vi "PS-RA01B FPGA.vi"() -> ()   [LabVIEW 2011]
uses:
  <vilib>/rvi/eio/common/nirviEmuTemplateMethod_errors.vi
  <vilib>/rvi/Memory/Memory_Emulation/niFpgaMemoryEmulationValidateCache.vi
  <vilib>/rvi/DataTransferAndStorage/Container/Common/niFpgaContainerGetUniqueNameForEmu.vi
  <vilib>/rvi/Memory/Memory_Emulation/nirvimemoryEmulationManagerCache_InsertValue.vi
  <vilib>/Utility/error.llb/Clear Errors.vi
  <vilib>/rvi/Memory/Memory_Emulation/nirvimemoryEmulationManagerCache_GetValue.vi
  <vilib>/rvi/Memory/Memory_Emulation/nirvimemoryEmulationManagerCache_SetValue.vi
  <vilib>/eio/EIONode/EIONode.xnode
  <vilib>/eio/EIOMethodNode/EIOMethodNode.xnode
  <vilib>/rvi/DataTransferAndStorage/Container/XNode/niFpgaContainer.xnode
  <vilib>/rvi/Memory/Memory_Emulation/nirvimemoryEmulation.vi
panel:
  out "ADDR":u8
  out "Mod6/AO1":fxp<+/-,20,5> format="%.17g"
  out "Mod2/AO3":fxp<+/-,20,5> format="%.17g"
  out "Mod2/AO2":fxp<+/-,20,5> format="%.17g"
  out "Mod2/AO1":fxp<+/-,20,5> format="%.17g"
  out "Mod2/AO0":fxp<+/-,20,5> format="%.17g"
  out "Mod6/AO3":fxp<+/-,20,5> format="%.17g"
  out "Mod6/AO2":fxp<+/-,20,5> format="%.17g"
  out "Mod6/AO0":fxp<+/-,20,5> format="%.17g"
  out "Timestamp":u32 caption="Tick Count(Ticks)"
  out "Mod5/AI0":fxp<+/-,20,5> format="%.17g"
  out "Mod5/AI2":fxp<+/-,20,5> format="%.17g"
  out "Mod5/AI3":fxp<+/-,20,5> format="%.17g"
  out "Mod1/AI0":fxp<+/-,20,5> format="%.17g"
  out "Mod1/AI1":fxp<+/-,20,5> format="%.17g"
  out "Mod1/AI2":fxp<+/-,20,5> format="%.17g"
  out "Mod1/AI3":fxp<+/-,20,5> format="%.17g"
  out "Mod5/AI1":fxp<+/-,20,5> format="%.17g"
  out "period":u32
  out "delay":u32
  out "dperiod":u32
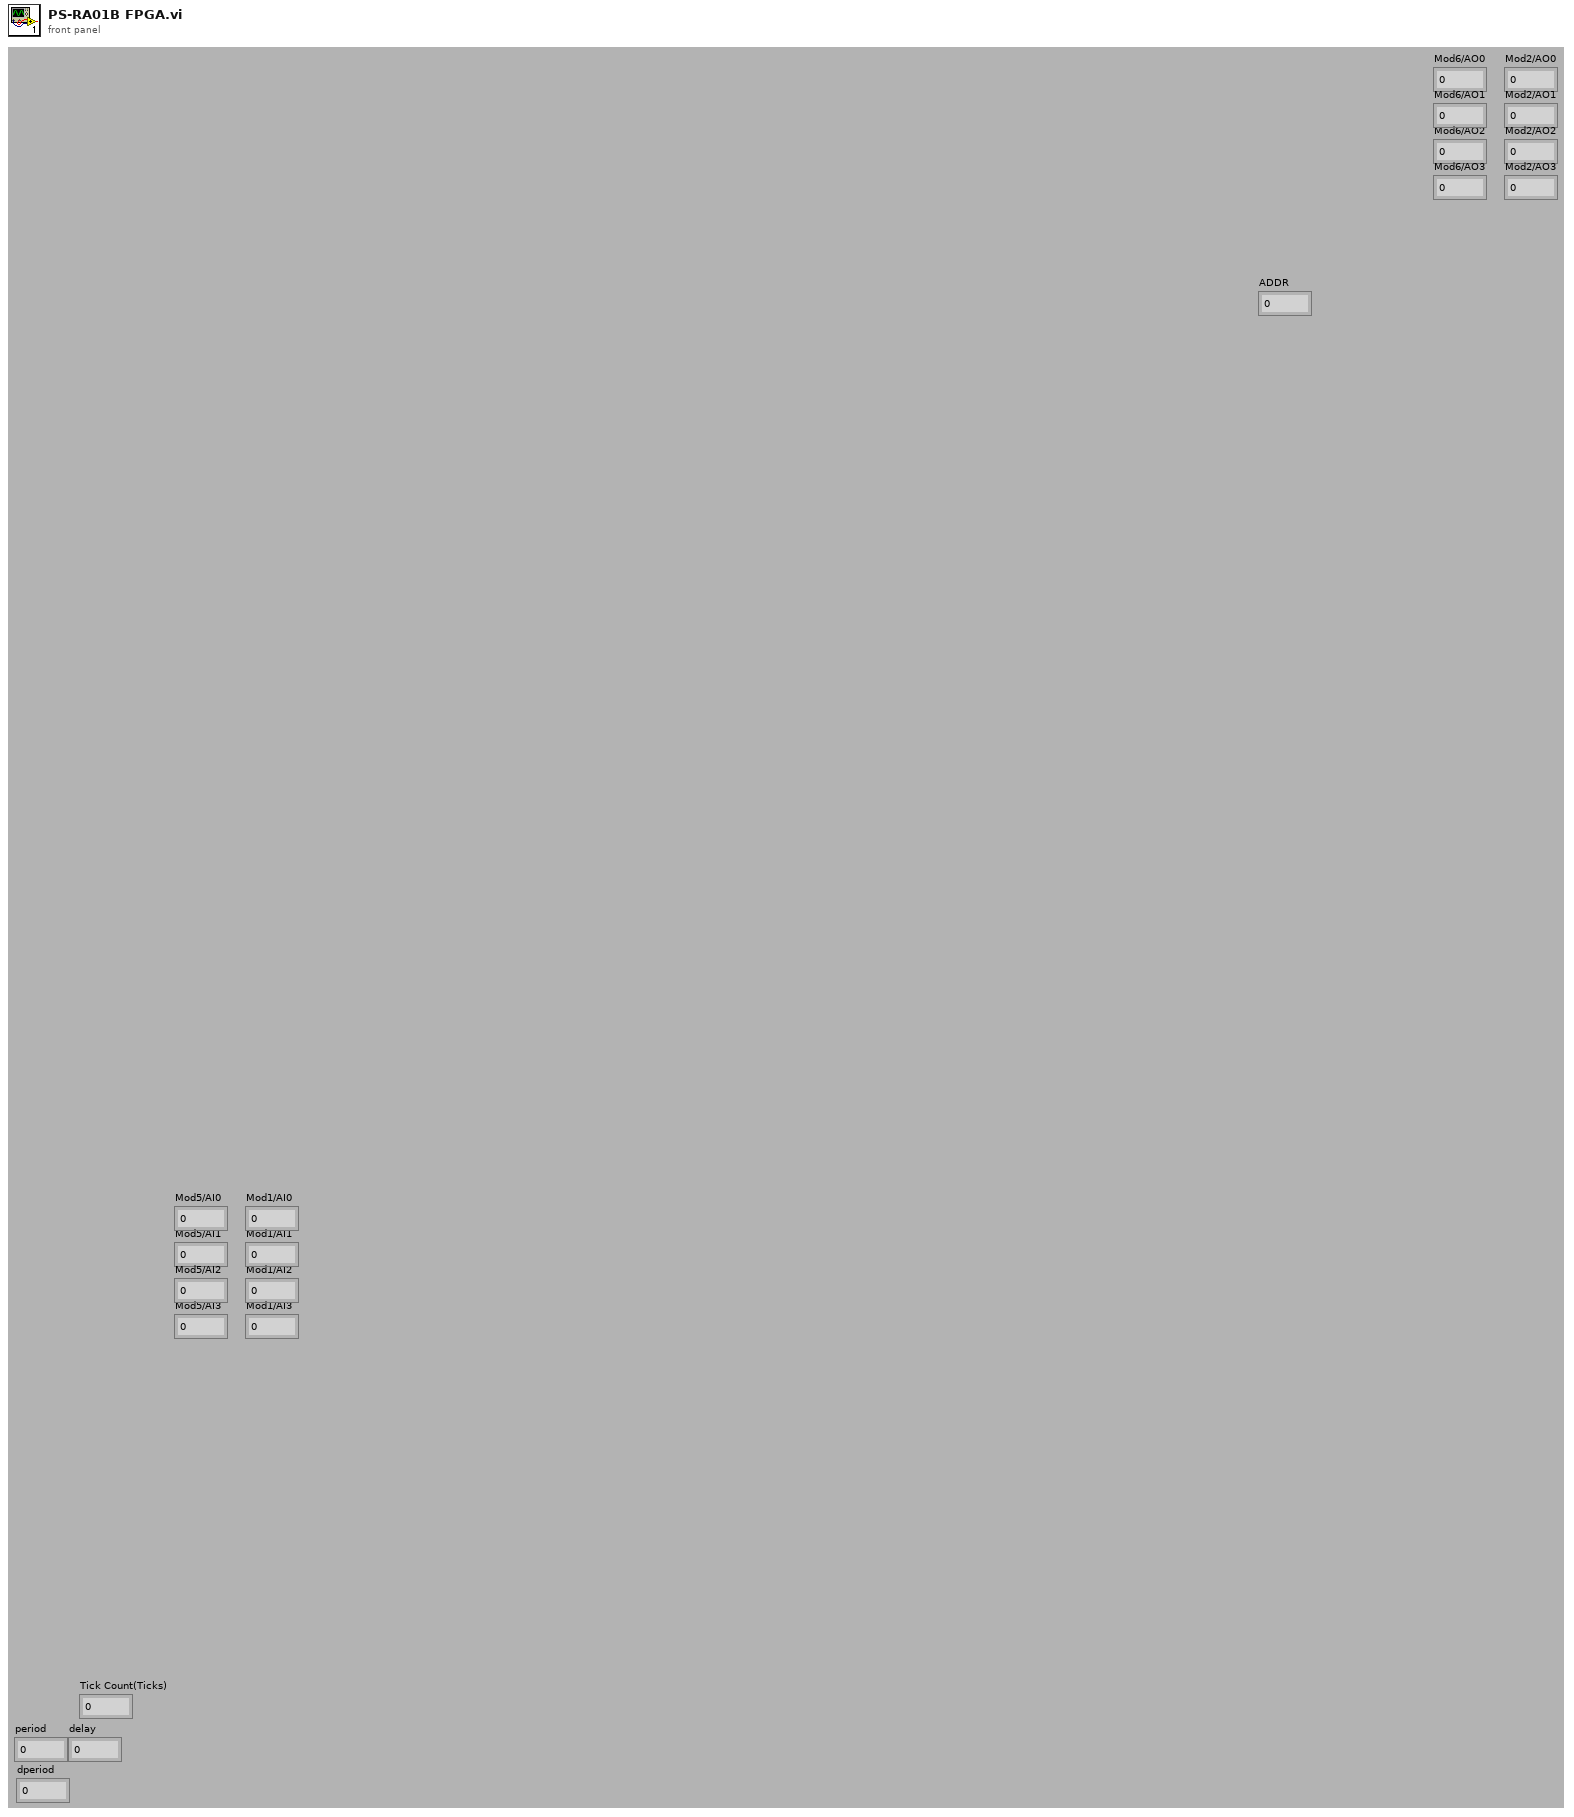
[diagram p1: front panel]
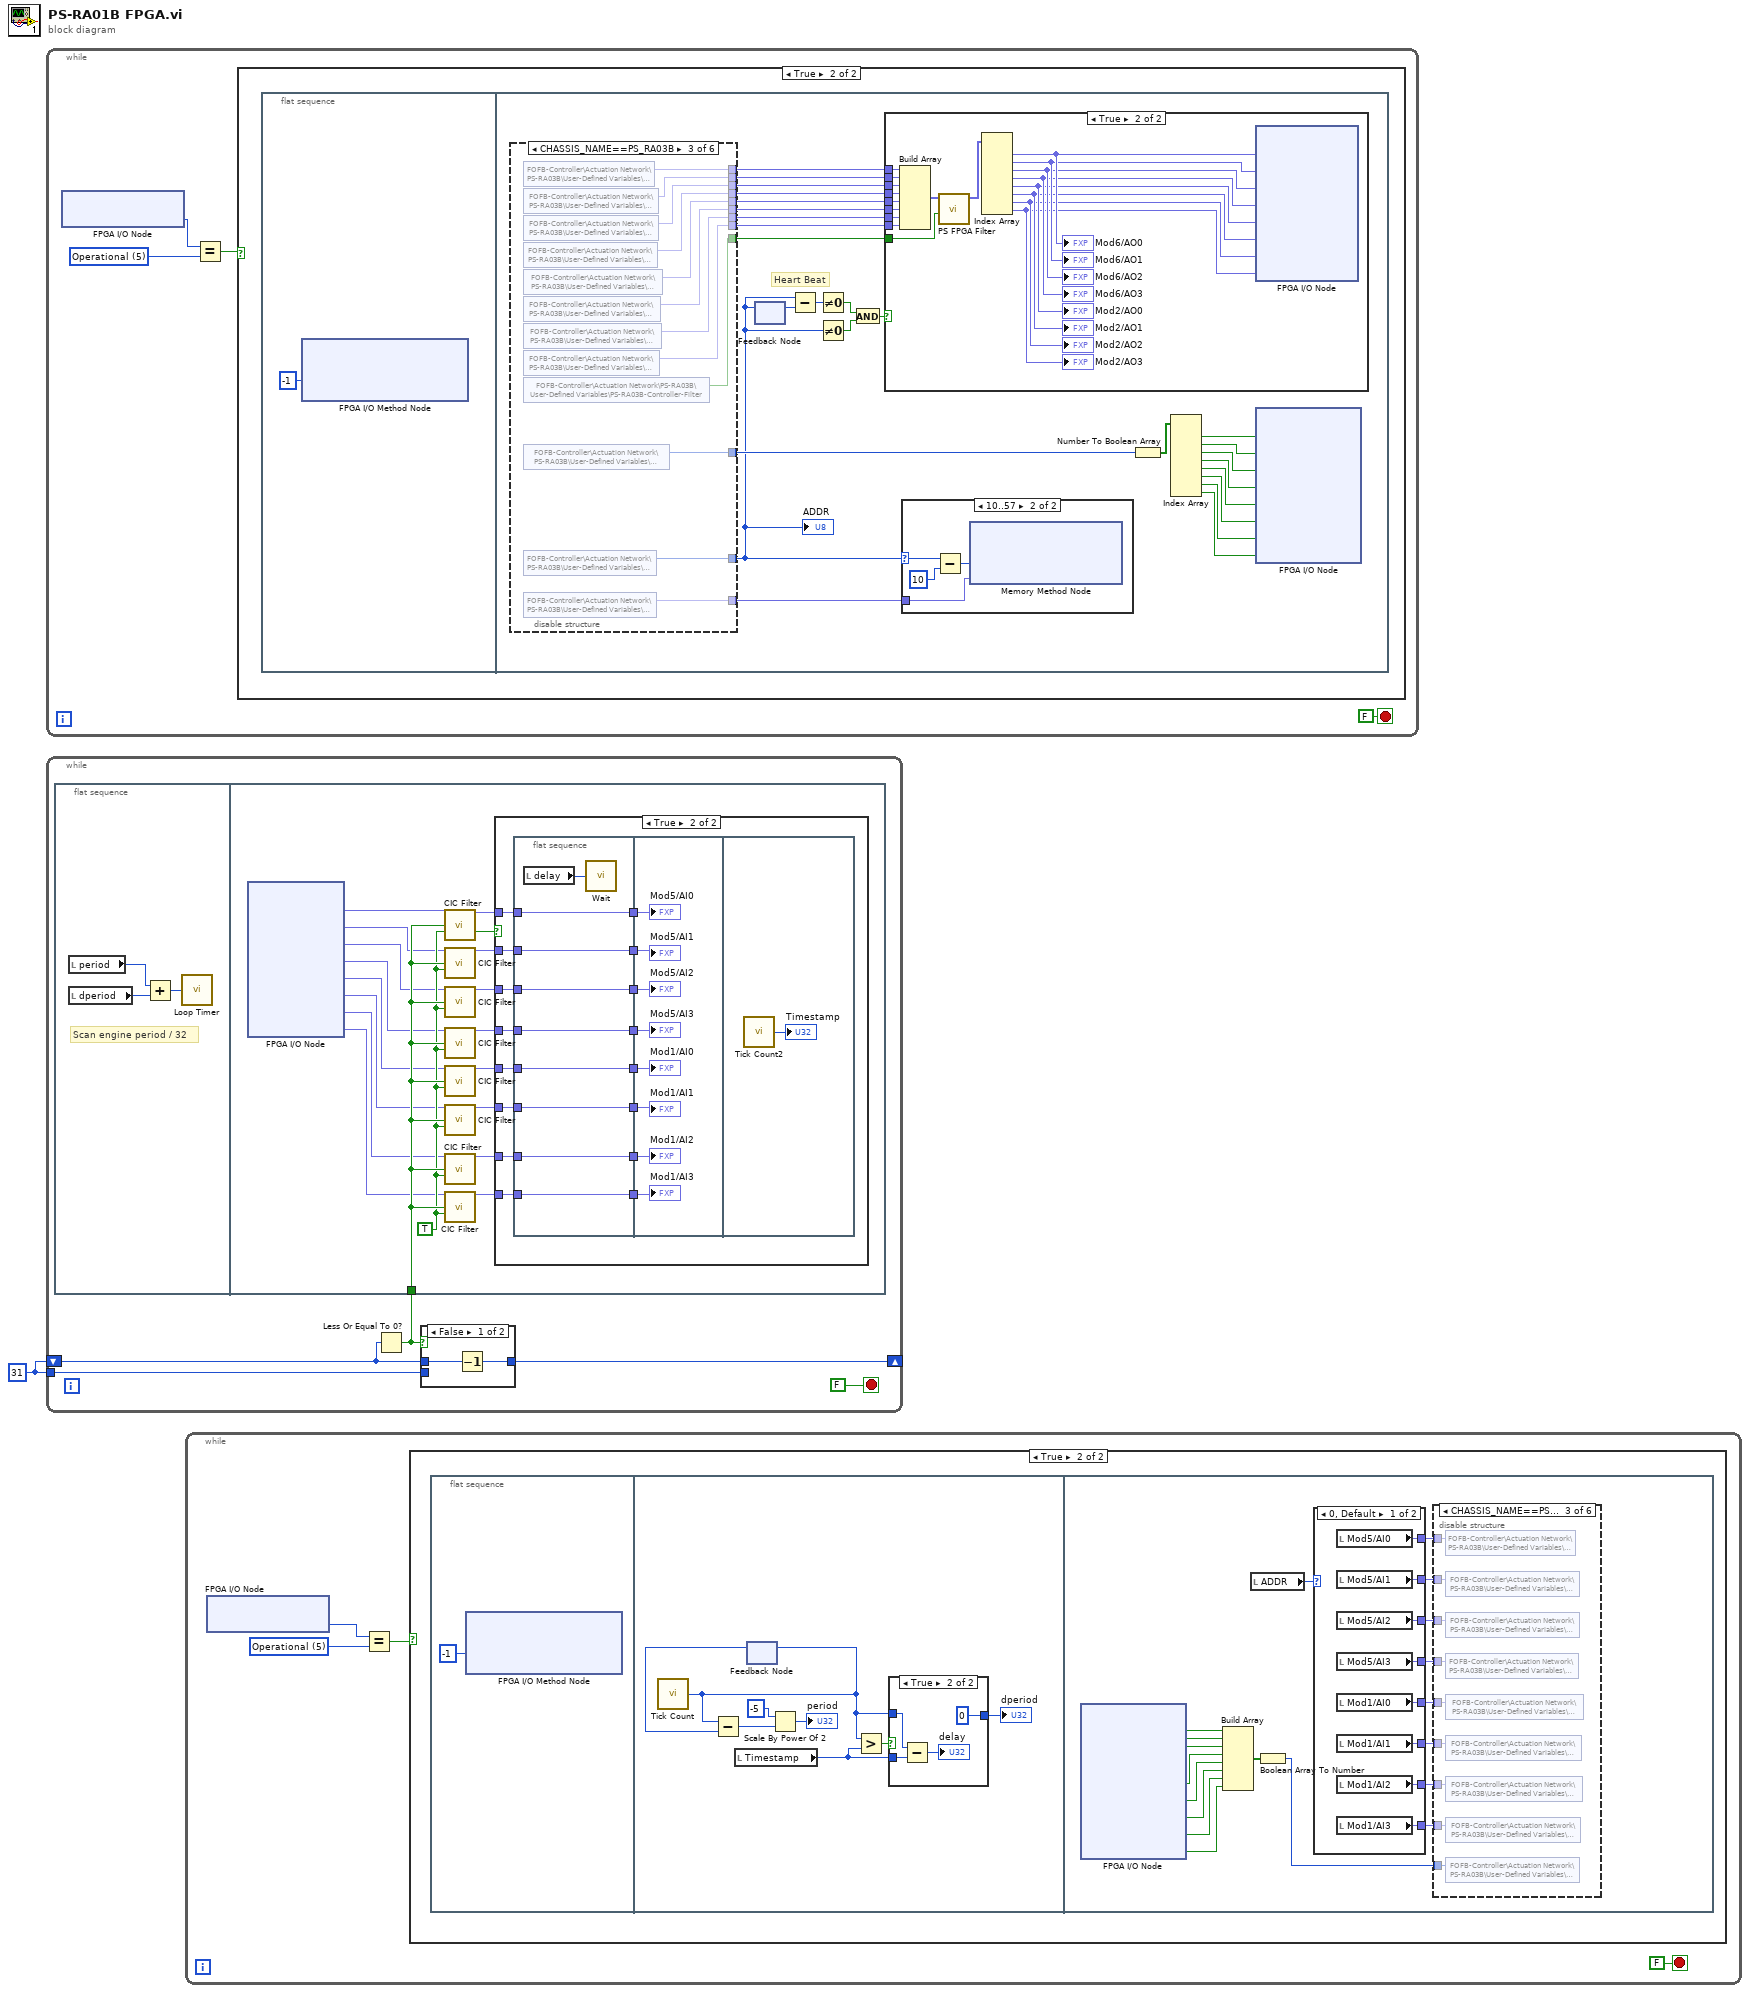
[diagram p0: block diagram]
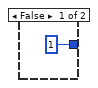
[diagram p5: hidden frame]
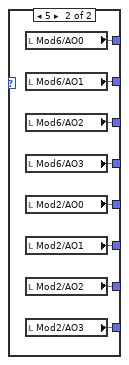
[diagram p6: hidden frame]
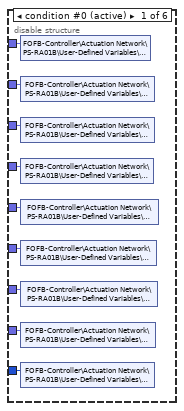
[diagram p7: hidden frame]
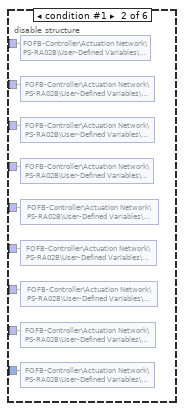
[diagram p8: hidden frame]
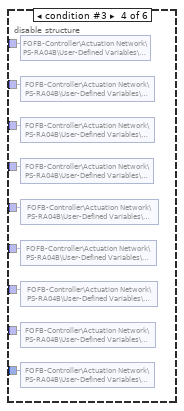
[diagram p9: hidden frame]
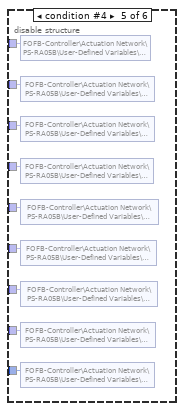
[diagram p10: hidden frame]
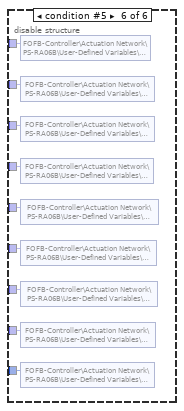
[diagram p11: hidden frame]
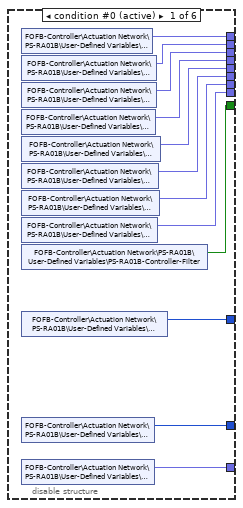
[diagram p15: hidden frame]
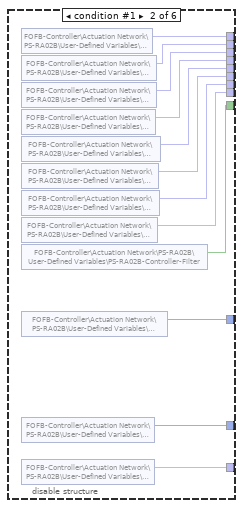
[diagram p16: hidden frame]
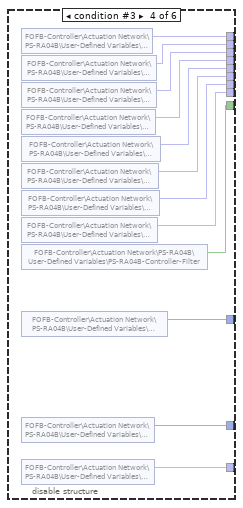
[diagram p17: hidden frame]
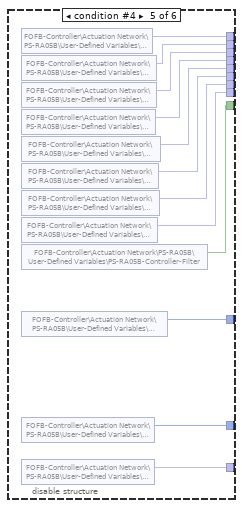
[diagram p18: hidden frame]
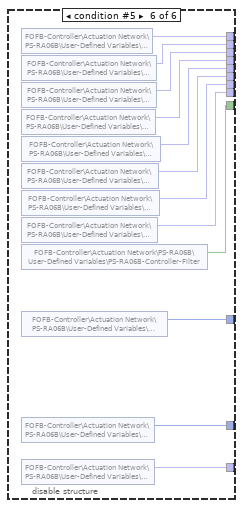
[diagram p19: hidden frame]
diagram:
  w1 = 31
  n1 = while {
    stop <- FALSE stop-if-true
    w2 = u8 5 items=["Init"=1, "PreOp"=2, "Bootstrap"=3, "SafeOp"=4, "Operational"=5]
    n2 = xnode "FPGA I/O Node"() -> ("EtherCAT State"=w3:u8)  [unwired: 1 in, 1 out]
    n3 = Equal?(x=w3, y=w2) -> (x = y?=w4:bool)
    n4 = case shown="True" w4 {
      frame False {
      }
      frame True {
        n5 = flat-sequence {
          frame #0 {
            n6 = xnode "FPGA I/O Method Node"("Timeout"=-1) -> ()  [unwired: 1 in, 2 out]
          }
          frame #1 {
            # "Heart Beat"
            n7 = disable-structure shown="CHASSIS_NAME==PS_RA03B" {
              disable-tunnel: [w67 w68 w81 w99 w111 w127] -> w32
              disable-tunnel: [w66 w69 w82 w98 w110 w122] -> w31
              disable-tunnel: [w65 w70 w83 w97 w109 w121] -> w30
              disable-tunnel: [w64 w71 w84 w96 w108 w120] -> w29
              disable-tunnel: [w63 w72 w85 w95 w107 w119] -> w28
              disable-tunnel: [w62 w73 w86 w94 w106 w118] -> w27
              disable-tunnel: [w61 w74 w87 w93 w105 w117] -> w26
              disable-tunnel: [w60 w75 w88 w92 w104 w116] -> w25
              disable-tunnel: [w59 w79 w91 w103 w115 w126] -> w12
              disable-tunnel: [w58 w78 w90 w102 w114 w125] -> w24
              disable-tunnel: [w57 w77 w89 w101 w113 w124] -> w22
              disable-tunnel: [w56 w76 w80 w100 w112 w123] -> w10
              frame condition #0 (active) {
                n8 = shared-variable "FOFB-Controller\\Actuation Network\\PS-RA01B\\User-Defined Variables\\ACH02-Setpoint"() -> (w67:fxp<+/-,20,5>)  [unwired: 1 in, 1 out]
                n9 = shared-variable "FOFB-Controller\\Actuation Network\\PS-RA01B\\User-Defined Variables\\RRA01B-Setpoint"() -> (w66:fxp<+/-,20,5>)  [unwired: 1 in, 1 out]
                n10 = shared-variable "FOFB-Controller\\Actuation Network\\PS-RA01B\\User-Defined Variables\\ALV02A-Setpoint"() -> (w65:fxp<+/-,20,5>)  [unwired: 1 in, 1 out]
                n11 = shared-variable "FOFB-Controller\\Actuation Network\\PS-RA01B\\User-Defined Variables\\ALV02B-Setpoint"() -> (w64:fxp<+/-,20,5>)  [unwired: 1 in, 1 out]
                n12 = shared-variable "FOFB-Controller\\Actuation Network\\PS-RA01B\\User-Defined Variables\\ACH03A-Setpoint"() -> (w63:fxp<+/-,20,5>)  [unwired: 1 in, 1 out]
                n13 = shared-variable "FOFB-Controller\\Actuation Network\\PS-RA01B\\User-Defined Variables\\ACV03A-Setpoint"() -> (w62:fxp<+/-,20,5>)  [unwired: 1 in, 1 out]
                n14 = shared-variable "FOFB-Controller\\Actuation Network\\PS-RA01B\\User-Defined Variables\\ACH01B-Setpoint"() -> (w61:fxp<+/-,20,5>)  [unwired: 1 in, 1 out]
                n15 = shared-variable "FOFB-Controller\\Actuation Network\\PS-RA01B\\User-Defined Variables\\ACV01B-Setpoint"() -> (w60:fxp<+/-,20,5>)  [unwired: 1 in, 1 out]
                n16 = shared-variable "FOFB-Controller\\Actuation Network\\PS-RA01B\\User-Defined Variables\\PS-RA01B-Controller-Filter"() -> (w58:bool)  [unwired: 1 in, 1 out]
                n17 = shared-variable "FOFB-Controller\\Actuation Network\\PS-RA01B\\User-Defined Variables\\PS-RA01B-ON-OFF"() -> (w59:u8)  [unwired: 1 in, 1 out]
                n18 = shared-variable "FOFB-Controller\\Actuation Network\\PS-RA01B\\User-Defined Variables\\PS-RA01B-ADDR"() -> (w56:u8)  [unwired: 1 in, 1 out]
                n19 = shared-variable "FOFB-Controller\\Actuation Network\\PS-RA01B\\User-Defined Variables\\PS-RA01B-DATA"() -> (w57:fxp<+/-,20,2>)  [unwired: 1 in, 1 out]
              }
              frame condition #1 {
                n20 = shared-variable "FOFB-Controller\\Actuation Network\\PS-RA02B\\User-Defined Variables\\ACH04-Setpoint"() -> (w68:fxp<+/-,20,5>)  [unwired: 1 in, 1 out]
                n21 = shared-variable "FOFB-Controller\\Actuation Network\\PS-RA02B\\User-Defined Variables\\RRA02B-Setpoint"() -> (w69:fxp<+/-,20,5>)  [unwired: 1 in, 1 out]
                n22 = shared-variable "FOFB-Controller\\Actuation Network\\PS-RA02B\\User-Defined Variables\\ALV04A-Setpoint"() -> (w70:fxp<+/-,20,5>)  [unwired: 1 in, 1 out]
                n23 = shared-variable "FOFB-Controller\\Actuation Network\\PS-RA02B\\User-Defined Variables\\ALV04B-Setpoint"() -> (w71:fxp<+/-,20,5>)  [unwired: 1 in, 1 out]
                n24 = shared-variable "FOFB-Controller\\Actuation Network\\PS-RA02B\\User-Defined Variables\\ACH05A-Setpoint"() -> (w72:fxp<+/-,20,5>)  [unwired: 1 in, 1 out]
                n25 = shared-variable "FOFB-Controller\\Actuation Network\\PS-RA02B\\User-Defined Variables\\ACV05A-Setpoint"() -> (w73:fxp<+/-,20,5>)  [unwired: 1 in, 1 out]
                n26 = shared-variable "FOFB-Controller\\Actuation Network\\PS-RA02B\\User-Defined Variables\\ACH03B-Setpoint"() -> (w74:fxp<+/-,20,5>)  [unwired: 1 in, 1 out]
                n27 = shared-variable "FOFB-Controller\\Actuation Network\\PS-RA02B\\User-Defined Variables\\ACV03B-Setpoint"() -> (w75:fxp<+/-,20,5>)  [unwired: 1 in, 1 out]
                n28 = shared-variable "FOFB-Controller\\Actuation Network\\PS-RA02B\\User-Defined Variables\\PS-RA02B-Controller-Filter"() -> (w78:bool)  [unwired: 1 in, 1 out]
                n29 = shared-variable "FOFB-Controller\\Actuation Network\\PS-RA02B\\User-Defined Variables\\PS-RA02B-ON-OFF"() -> (w79:u8)  [unwired: 1 in, 1 out]
                n30 = shared-variable "FOFB-Controller\\Actuation Network\\PS-RA02B\\User-Defined Variables\\PS-RA02B-ADDR"() -> (w76:u8)  [unwired: 1 in, 1 out]
                n31 = shared-variable "FOFB-Controller\\Actuation Network\\PS-RA02B\\User-Defined Variables\\PS-RA02B-DATA"() -> (w77:fxp<+/-,20,2>)  [unwired: 1 in, 1 out]
              }
              frame condition #2 {
                n32 = shared-variable "FOFB-Controller\\Actuation Network\\PS-RA03B\\User-Defined Variables\\ACH06-Setpoint"() -> (w81:fxp<+/-,20,5>)  [unwired: 1 in, 1 out]
                n33 = shared-variable "FOFB-Controller\\Actuation Network\\PS-RA03B\\User-Defined Variables\\RRA03B-Setpoint"() -> (w82:fxp<+/-,20,5>)  [unwired: 1 in, 1 out]
                n34 = shared-variable "FOFB-Controller\\Actuation Network\\PS-RA03B\\User-Defined Variables\\ALV06A-Setpoint"() -> (w83:fxp<+/-,20,5>)  [unwired: 1 in, 1 out]
                n35 = shared-variable "FOFB-Controller\\Actuation Network\\PS-RA03B\\User-Defined Variables\\ALV06B-Setpoint"() -> (w84:fxp<+/-,20,5>)  [unwired: 1 in, 1 out]
                n36 = shared-variable "FOFB-Controller\\Actuation Network\\PS-RA03B\\User-Defined Variables\\ACH07A-Setpoint"() -> (w85:fxp<+/-,20,5>)  [unwired: 1 in, 1 out]
                n37 = shared-variable "FOFB-Controller\\Actuation Network\\PS-RA03B\\User-Defined Variables\\ACV07A-Setpoint"() -> (w86:fxp<+/-,20,5>)  [unwired: 1 in, 1 out]
                n38 = shared-variable "FOFB-Controller\\Actuation Network\\PS-RA03B\\User-Defined Variables\\ACH05B-Setpoint"() -> (w87:fxp<+/-,20,5>)  [unwired: 1 in, 1 out]
                n39 = shared-variable "FOFB-Controller\\Actuation Network\\PS-RA03B\\User-Defined Variables\\ACV05B-Setpoint"() -> (w88:fxp<+/-,20,5>)  [unwired: 1 in, 1 out]
                n40 = shared-variable "FOFB-Controller\\Actuation Network\\PS-RA03B\\User-Defined Variables\\PS-RA03B-Controller-Filter"() -> (w90:bool)  [unwired: 1 in, 1 out]
                n41 = shared-variable "FOFB-Controller\\Actuation Network\\PS-RA03B\\User-Defined Variables\\PS-RA03B-ON-OFF"() -> (w91:u8)  [unwired: 1 in, 1 out]
                n42 = shared-variable "FOFB-Controller\\Actuation Network\\PS-RA03B\\User-Defined Variables\\PS-RA03B-ADDR"() -> (w80:u8)  [unwired: 1 in, 1 out]
                n43 = shared-variable "FOFB-Controller\\Actuation Network\\PS-RA03B\\User-Defined Variables\\PS-RA03B-DATA"() -> (w89:fxp<+/-,20,2>)  [unwired: 1 in, 1 out]
              }
              frame condition #3 {
                n44 = shared-variable "FOFB-Controller\\Actuation Network\\PS-RA04B\\User-Defined Variables\\ACH08-Setpoint"() -> (w99:fxp<+/-,20,5>)  [unwired: 1 in, 1 out]
                n45 = shared-variable "FOFB-Controller\\Actuation Network\\PS-RA04B\\User-Defined Variables\\RRA04B-Setpoint"() -> (w98:fxp<+/-,20,5>)  [unwired: 1 in, 1 out]
                n46 = shared-variable "FOFB-Controller\\Actuation Network\\PS-RA04B\\User-Defined Variables\\ALV08A-Setpoint"() -> (w97:fxp<+/-,20,5>)  [unwired: 1 in, 1 out]
                n47 = shared-variable "FOFB-Controller\\Actuation Network\\PS-RA04B\\User-Defined Variables\\ALV08B-Setpoint"() -> (w96:fxp<+/-,20,5>)  [unwired: 1 in, 1 out]
                n48 = shared-variable "FOFB-Controller\\Actuation Network\\PS-RA04B\\User-Defined Variables\\ACH09A-Setpoint"() -> (w95:fxp<+/-,20,5>)  [unwired: 1 in, 1 out]
                n49 = shared-variable "FOFB-Controller\\Actuation Network\\PS-RA04B\\User-Defined Variables\\ACV09A-Setpoint"() -> (w94:fxp<+/-,20,5>)  [unwired: 1 in, 1 out]
                n50 = shared-variable "FOFB-Controller\\Actuation Network\\PS-RA04B\\User-Defined Variables\\ACH07B-Setpoint"() -> (w93:fxp<+/-,20,5>)  [unwired: 1 in, 1 out]
                n51 = shared-variable "FOFB-Controller\\Actuation Network\\PS-RA04B\\User-Defined Variables\\ACV07B-Setpoint"() -> (w92:fxp<+/-,20,5>)  [unwired: 1 in, 1 out]
                n52 = shared-variable "FOFB-Controller\\Actuation Network\\PS-RA04B\\User-Defined Variables\\PS-RA04B-Controller-Filter"() -> (w102:bool)  [unwired: 1 in, 1 out]
                n53 = shared-variable "FOFB-Controller\\Actuation Network\\PS-RA04B\\User-Defined Variables\\PS-RA04B-ON-OFF"() -> (w103:u8)  [unwired: 1 in, 1 out]
                n54 = shared-variable "FOFB-Controller\\Actuation Network\\PS-RA04B\\User-Defined Variables\\PS-RA04B-ADDR"() -> (w100:u8)  [unwired: 1 in, 1 out]
                n55 = shared-variable "FOFB-Controller\\Actuation Network\\PS-RA04B\\User-Defined Variables\\PS-RA04B-DATA"() -> (w101:fxp<+/-,20,2>)  [unwired: 1 in, 1 out]
              }
              frame condition #4 {
                n56 = shared-variable "FOFB-Controller\\Actuation Network\\PS-RA05B\\User-Defined Variables\\ACH10-Setpoint"() -> (w111:fxp<+/-,20,5>)  [unwired: 1 in, 1 out]
                n57 = shared-variable "FOFB-Controller\\Actuation Network\\PS-RA05B\\User-Defined Variables\\RRA05B-Setpoint"() -> (w110:fxp<+/-,20,5>)  [unwired: 1 in, 1 out]
                n58 = shared-variable "FOFB-Controller\\Actuation Network\\PS-RA05B\\User-Defined Variables\\ALV10A-Setpoint"() -> (w109:fxp<+/-,20,5>)  [unwired: 1 in, 1 out]
                n59 = shared-variable "FOFB-Controller\\Actuation Network\\PS-RA05B\\User-Defined Variables\\ALV10B-Setpoint"() -> (w108:fxp<+/-,20,5>)  [unwired: 1 in, 1 out]
                n60 = shared-variable "FOFB-Controller\\Actuation Network\\PS-RA05B\\User-Defined Variables\\ACH11A-Setpoint"() -> (w107:fxp<+/-,20,5>)  [unwired: 1 in, 1 out]
                n61 = shared-variable "FOFB-Controller\\Actuation Network\\PS-RA05B\\User-Defined Variables\\ACV11A-Setpoint"() -> (w106:fxp<+/-,20,5>)  [unwired: 1 in, 1 out]
                n62 = shared-variable "FOFB-Controller\\Actuation Network\\PS-RA05B\\User-Defined Variables\\ACH09B-Setpoint"() -> (w105:fxp<+/-,20,5>)  [unwired: 1 in, 1 out]
                n63 = shared-variable "FOFB-Controller\\Actuation Network\\PS-RA05B\\User-Defined Variables\\ACV09B-Setpoint"() -> (w104:fxp<+/-,20,5>)  [unwired: 1 in, 1 out]
                n64 = shared-variable "FOFB-Controller\\Actuation Network\\PS-RA05B\\User-Defined Variables\\PS-RA05B-Controller-Filter"() -> (w114:bool)  [unwired: 1 in, 1 out]
                n65 = shared-variable "FOFB-Controller\\Actuation Network\\PS-RA05B\\User-Defined Variables\\PS-RA05B-ON-OFF"() -> (w115:u8)  [unwired: 1 in, 1 out]
                n66 = shared-variable "FOFB-Controller\\Actuation Network\\PS-RA05B\\User-Defined Variables\\PS-RA05B-ADDR"() -> (w112:u8)  [unwired: 1 in, 1 out]
                n67 = shared-variable "FOFB-Controller\\Actuation Network\\PS-RA05B\\User-Defined Variables\\PS-RA05B-DATA"() -> (w113:fxp<+/-,20,2>)  [unwired: 1 in, 1 out]
              }
              frame condition #5 {
                n68 = shared-variable "FOFB-Controller\\Actuation Network\\PS-RA06B\\User-Defined Variables\\ACH12-Setpoint"() -> (w127:fxp<+/-,20,5>)  [unwired: 1 in, 1 out]
                n69 = shared-variable "FOFB-Controller\\Actuation Network\\PS-RA06B\\User-Defined Variables\\RRA06B-Setpoint"() -> (w122:fxp<+/-,20,5>)  [unwired: 1 in, 1 out]
                n70 = shared-variable "FOFB-Controller\\Actuation Network\\PS-RA06B\\User-Defined Variables\\ALV12A-Setpoint"() -> (w121:fxp<+/-,20,5>)  [unwired: 1 in, 1 out]
                n71 = shared-variable "FOFB-Controller\\Actuation Network\\PS-RA06B\\User-Defined Variables\\ALV12B-Setpoint"() -> (w120:fxp<+/-,20,5>)  [unwired: 1 in, 1 out]
                n72 = shared-variable "FOFB-Controller\\Actuation Network\\PS-RA06B\\User-Defined Variables\\ACH01A-Setpoint"() -> (w119:fxp<+/-,20,5>)  [unwired: 1 in, 1 out]
                n73 = shared-variable "FOFB-Controller\\Actuation Network\\PS-RA06B\\User-Defined Variables\\ACV01A-Setpoint"() -> (w118:fxp<+/-,20,5>)  [unwired: 1 in, 1 out]
                n74 = shared-variable "FOFB-Controller\\Actuation Network\\PS-RA06B\\User-Defined Variables\\ACH11B-Setpoint"() -> (w117:fxp<+/-,20,5>)  [unwired: 1 in, 1 out]
                n75 = shared-variable "FOFB-Controller\\Actuation Network\\PS-RA06B\\User-Defined Variables\\ACV11B-Setpoint"() -> (w116:fxp<+/-,20,5>)  [unwired: 1 in, 1 out]
                n76 = shared-variable "FOFB-Controller\\Actuation Network\\PS-RA06B\\User-Defined Variables\\PS-RA06B-Controller-Filter"() -> (w125:bool)  [unwired: 1 in, 1 out]
                n77 = shared-variable "FOFB-Controller\\Actuation Network\\PS-RA06B\\User-Defined Variables\\PS-RA06B-ON-OFF"() -> (w126:u8)  [unwired: 1 in, 1 out]
                n78 = shared-variable "FOFB-Controller\\Actuation Network\\PS-RA06B\\User-Defined Variables\\PS-RA06B-ADDR"() -> (w123:u8)  [unwired: 1 in, 1 out]
                n79 = shared-variable "FOFB-Controller\\Actuation Network\\PS-RA06B\\User-Defined Variables\\PS-RA06B-DATA"() -> (w124:fxp<+/-,20,2>)  [unwired: 1 in, 1 out]
              }
            }
            "ADDR" <- w10
            n80 = feedback #1() -> (w23:u8)  [unwired: 1 in]
            n81 = feedback-in #1(w10) -> ()
            n82 = Subtract(x=w10, y=w23) -> (x-y=w11:i8)
            n83 = Not Equal To 0?(x=w11) -> (x != 0?=w9:bool)
            n84 = Not Equal To 0?(x=w10) -> (x != 0?=w8:bool)
            n85 = And(x=w9, y=w8) -> (x .and. y?=w7:bool)
            n86 = case shown="True" w7 {
              tunnel: w32 -> [_ w55]
              tunnel: w31 -> [_ w54]
              tunnel: w30 -> [_ w53]
              tunnel: w29 -> [_ w52]
              tunnel: w28 -> [_ w51]
              tunnel: w27 -> [_ w50]
              tunnel: w26 -> [_ w49]
              tunnel: w25 -> [_ w48]
              tunnel: w24 -> [_ w45]
              frame False {
              }
              frame True {
                n87 = Build Array(w55, w54, w53, w52, w51, w50, w49, w48) -> (w47:fxp<+/-,20,5>[])
                n88 = call "PS FPGA Filter.vi"("loop?"=w45, "input"=w47) -> ("output"=w46:fxp<+/-,20,5>[])  [unwired: 9 in]
                n89 = Index Array(array=w46) -> (element #1=w44:fxp<+/-,20,5>, element #2=w43:fxp<+/-,20,5>, element #3=w42:fxp<+/-,20,5>, element #4=w41:fxp<+/-,20,5>, element #5=w40:fxp<+/-,20,5>, element #6=w39:fxp<+/-,20,5>, element #7=w38:fxp<+/-,20,5>, element #8=w37:fxp<+/-,20,5>)  [unwired: 8 in]
                "Mod6/AO0" <- w44
                "Mod6/AO2" <- w42
                "Mod6/AO3" <- w41
                "Mod2/AO0" <- w40
                "Mod2/AO1" <- w39
                "Mod2/AO2" <- w38
                "Mod2/AO3" <- w37
                "Mod6/AO1" <- w43
                n90 = xnode "FPGA I/O Node"("Mod6/AO0"=w44, "Mod6/AO1"=w43, "Mod6/AO2"=w42, "Mod6/AO3"=w41, "Mod2/AO0"=w40, "Mod2/AO1"=w39, "Mod2/AO2"=w38, "Mod2/AO3"=w37) -> ()  [unwired: 8 in, 8 out]
              }
            }
            n91 = case shown="10..57" w10 {
              selector: w10 -> [_ w36]
              tunnel: w22 -> [_ w33]
              frame 0, Default {
              }
              frame 10..57 {
                n92 = Subtract(x=w36, y=u8 10) -> (x-y=w34:u8)
                n93 = xnode ("Memory Method Node")("Address"=w34, "Data"=w33) -> ()  [unwired: 1 in, 1 out]
              }
            }
            n94 = Number To Boolean Array(number=w12) -> (Boolean array=w21:bool[])
            n95 = Index Array(array=w21) -> (element #1=w13:bool, element #2=w14:bool, element #3=w15:bool, element #4=w16:bool, element #5=w17:bool, element #6=w18:bool, element #7=w19:bool, element #8=w20:bool)  [unwired: 8 in]
            n96 = xnode "FPGA I/O Node"("Mod4/DIO6"=w13, "Mod4/DIO7"=w14, "Mod4/DIO4"=w15, "Mod4/DIO5"=w16, "Mod4/DIO2"=w17, "Mod4/DIO3"=w18, "Mod4/DIO0"=w19, "Mod4/DIO1"=w20) -> ()  [unwired: 8 in, 8 out]
          }
        }
      }
    }
  }
  n97 = while {
    shift-right: [w131] -> _
    shift-left: w1 -> [w130]
    tunnel: w1 -> [w128]
    stop <- FALSE stop-if-true
    n98 = flat-sequence {
      tunnel: w129 -> [w157]
      frame #0 {
        # "Scan engine period / 32"
        n99 = local read "period"() -> (w138:u32)
        n100 = local read "dperiod"() -> (w137:u32)
        n101 = Add(x=w138, y=w137) -> (x+y=w136:u32)
        n102 = call "Loop Timer"("Count(Ticks)"=w136) -> ()  [unwired: 1 out]
      }
      frame #1 {
        w156 = TRUE ("input valid")
        n103 = xnode "FPGA I/O Node"() -> ("Mod5/AI0"=w155:fxp<+/-,20,5>, "Mod5/AI1"=w154:fxp<+/-,20,5>, "Mod5/AI2"=w153:fxp<+/-,20,5>, "Mod5/AI3"=w152:fxp<+/-,20,5>, "Mod1/AI0"=w151:fxp<+/-,20,5>, "Mod1/AI1"=w150:fxp<+/-,20,5>, "Mod1/AI2"=w149:fxp<+/-,20,5>, "Mod1/AI3"=w148:fxp<+/-,20,5>)  [unwired: 8 in, 8 out]
        n104 = call "CIC Filter.vi"("input data"=w155, "sample"=w157, "input valid"=w156) -> ("output data"=w146:fxp<+/-,20,5>, "output valid"=w147:bool)  [unwired: 10 in, 1 out]
        n105 = call "CIC Filter.vi"("input data"=w154, "sample"=w157, "input valid"=w156) -> ("output data"=w145:fxp<+/-,20,5>)  [unwired: 10 in, 2 out]
        n106 = call "CIC Filter.vi"("input data"=w153, "sample"=w157, "input valid"=w156) -> ("output data"=w144:fxp<+/-,20,5>)  [unwired: 10 in, 2 out]
        n107 = call "CIC Filter.vi"("input data"=w152, "sample"=w157, "input valid"=w156) -> ("output data"=w143:fxp<+/-,20,5>)  [unwired: 10 in, 2 out]
        n108 = call "CIC Filter.vi"("input data"=w151, "sample"=w157, "input valid"=w156) -> ("output data"=w142:fxp<+/-,20,5>)  [unwired: 10 in, 2 out]
        n109 = call "CIC Filter.vi"("input data"=w150, "sample"=w157, "input valid"=w156) -> ("output data"=w141:fxp<+/-,20,5>)  [unwired: 10 in, 2 out]
        n110 = call "CIC Filter.vi"("input data"=w149, "sample"=w157, "input valid"=w156) -> ("output data"=w140:fxp<+/-,20,5>)  [unwired: 10 in, 2 out]
        n111 = call "CIC Filter.vi"("input data"=w148, "sample"=w157, "input valid"=w156) -> ("output data"=w139:fxp<+/-,20,5>)  [unwired: 10 in, 2 out]
        n112 = case shown="True" w147 {
          tunnel: w146 -> [_ w173]
          tunnel: w145 -> [_ w171]
          tunnel: w144 -> [_ w169]
          tunnel: w143 -> [_ w168]
          tunnel: w142 -> [_ w165]
          tunnel: w141 -> [_ w163]
          tunnel: w140 -> [_ w161]
          tunnel: w139 -> [_ w159]
          frame False {
          }
          frame True {
            n113 = flat-sequence {
              tunnel: w173 -> [w182]
              tunnel: [w182] -> w172
              tunnel: w171 -> [w180]
              tunnel: [w180] -> w170
              tunnel: w169 -> [w178]
              tunnel: w168 -> [w179]
              tunnel: [w179] -> w167
              tunnel: [w178] -> w166
              tunnel: w165 -> [w177]
              tunnel: [w177] -> w164
              tunnel: w163 -> [w176]
              tunnel: [w176] -> w162
              tunnel: w161 -> [w175]
              tunnel: [w175] -> w160
              tunnel: w159 -> [w174]
              tunnel: [w174] -> w158
              tunnel: w172 -> [w189]
              tunnel: w170 -> [w190]
              tunnel: w167 -> [w188]
              tunnel: w166 -> [w187]
              tunnel: w164 -> [w186]
              tunnel: w162 -> [w185]
              tunnel: w160 -> [w184]
              tunnel: w158 -> [w183]
              frame #0 {
                n114 = local read "delay"() -> (w181:u32)
                n115 = call "Wait"("Count(Ticks)"=w181) -> ()  [unwired: 1 out]
              }
              frame #1 {
                "Mod5/AI0" <- w189
                "Mod5/AI2" <- w187
                "Mod5/AI3" <- w188
                "Mod1/AI0" <- w186
                "Mod1/AI1" <- w185
                "Mod1/AI2" <- w184
                "Mod1/AI3" <- w183
                "Mod5/AI1" <- w190
              }
              frame #2 {
                n116 = call "Tick Count2"() -> ("Tick Count(Ticks)"=→"Timestamp":u32)
              }
            }
          }
        }
      }
    }
    n117 = Less Or Equal To 0?(x=w130) -> (x <= 0?=w129:bool)
    n118 = case shown="False" w129 {
      tunnel: [w134 w135] -> w131
      tunnel: w130 -> [w133 _]
      tunnel: w128 -> [_ w135]
      frame False {
        n119 = Decrement(x=w133) -> (x-1=w134:i32)
      }
      frame True {
      }
    }
  }
  n120 = while {
    stop <- FALSE stop-if-true
    w194 = u8 5 items=["Init"=1, "PreOp"=2, "Bootstrap"=3, "SafeOp"=4, "Operational"=5]
    n121 = xnode "FPGA I/O Node"() -> ("EtherCAT State"=w193:u8)  [unwired: 1 in, 1 out]
    n122 = Equal?(x=w193, y=w194) -> (x = y?=w192:bool)
    n123 = case shown="True" w192 {
      frame False {
      }
      frame True {
        n124 = flat-sequence {
          frame #0 {
            n125 = xnode "FPGA I/O Method Node"("Timeout"=-1) -> ()  [unwired: 1 in, 2 out]
          }
          frame #1 {
            n126 = call "Tick Count"() -> ("Tick Count(Ticks)"=w198:u32)
            n127 = local read "Timestamp"() -> (w200:u32)
            n128 = feedback #2() -> (w197:u32)  [unwired: 1 in]
            n129 = Subtract(x=w198, y=w197) -> (x-y=w203:u32)
            n130 = feedback-in #2(w198) -> ()
            n131 = Scale By Power Of 2(n=i8 -5, x=w203) -> (x*2^n=→"period":u32)
            n132 = Greater?(x=w198, y=w200) -> (0:w201:bool)
            n133 = case shown="True" w201 {
              tunnel: w198 -> [_ w209]
              tunnel: w200 -> [_ w208]
              tunnel: [u32 1 ("dt 2") u32 0 ("dt 2")] -> w199
              frame False {
              }
              frame True {
                n134 = Subtract(x=w209, y=w208) -> (x-y=→"delay":u32)
              }
            }
            "dperiod" <- w199
          }
          frame #2 {
            n135 = xnode "FPGA I/O Node"() -> ("Mod3/DIO6"=w213:bool, "Mod3/DIO7"=w214:bool, "Mod3/DIO4"=w215:bool, "Mod3/DIO5"=w216:bool, "Mod3/DIO2"=w217:bool, "Mod3/DIO3"=w218:bool, "Mod3/DIO0"=w219:bool, "Mod3/DIO1"=w220:bool)  [unwired: 8 in, 8 out]
            n136 = Build Array(w213, w214, w215, w216, w217, w218, w219, w220) -> (w212:bool[])
            n137 = local read "ADDR"() -> (w210:u8)
            n138 = Boolean Array To Number(Boolean array=w212) -> (number=w211:u8)
            n139 = case shown="0, Default" w210 {
              tunnel: [w236 w244] -> w228
              tunnel: [w235 w243] -> w227
              tunnel: [w234 w242] -> w226
              tunnel: [w233 w237] -> w225
              tunnel: [w232 w238] -> w224
              tunnel: [w231 w239] -> w223
              tunnel: [w230 w240] -> w222
              tunnel: [w229 w241] -> w221
              frame 0, Default {
                n140 = local read "Mod5/AI0"() -> (w236:fxp<+/-,20,5>)
                n141 = local read "Mod5/AI1"() -> (w235:fxp<+/-,20,5>)
                n142 = local read "Mod5/AI2"() -> (w234:fxp<+/-,20,5>)
                n143 = local read "Mod5/AI3"() -> (w233:fxp<+/-,20,5>)
                n144 = local read "Mod1/AI0"() -> (w232:fxp<+/-,20,5>)
                n145 = local read "Mod1/AI1"() -> (w231:fxp<+/-,20,5>)
                n146 = local read "Mod1/AI2"() -> (w230:fxp<+/-,20,5>)
                n147 = local read "Mod1/AI3"() -> (w229:fxp<+/-,20,5>)
              }
              frame 5 {
                n148 = local read "Mod6/AO0"() -> (w244:fxp<+/-,20,5>)
                n149 = local read "Mod6/AO1"() -> (w243:fxp<+/-,20,5>)
                n150 = local read "Mod6/AO2"() -> (w242:fxp<+/-,20,5>)
                n151 = local read "Mod6/AO3"() -> (w237:fxp<+/-,20,5>)
                n152 = local read "Mod2/AO0"() -> (w238:fxp<+/-,20,5>)
                n153 = local read "Mod2/AO1"() -> (w239:fxp<+/-,20,5>)
                n154 = local read "Mod2/AO2"() -> (w240:fxp<+/-,20,5>)
                n155 = local read "Mod2/AO3"() -> (w241:fxp<+/-,20,5>)
              }
            }
            n156 = disable-structure shown="CHASSIS_NAME==PS_RA03B" {
              disable-tunnel: w228 -> [w253 w261 w270 w279 w288 w297]
              disable-tunnel: w227 -> [w252 w260 w269 w278 w287 w296]
              disable-tunnel: w226 -> [w251 w259 w268 w277 w286 w295]
              disable-tunnel: w225 -> [w250 w258 w267 w276 w285 w294]
              disable-tunnel: w224 -> [w249 w257 w266 w275 w284 w293]
              disable-tunnel: w223 -> [w248 w256 w265 w274 w283 w292]
              disable-tunnel: w222 -> [w247 w255 w264 w273 w282 w291]
              disable-tunnel: w221 -> [w246 w254 w263 w272 w281 w290]
              disable-tunnel: w211 -> [w245 w262 w271 w280 w289 w298]
              frame condition #0 (active) {
                n157 = shared-variable "FOFB-Controller\\Actuation Network\\PS-RA01B\\User-Defined Variables\\ACH02-Reading"(w253) -> ()  [unwired: 1 in, 1 out]
                n158 = shared-variable "FOFB-Controller\\Actuation Network\\PS-RA01B\\User-Defined Variables\\RRA01B-Reading"(w252) -> ()  [unwired: 1 in, 1 out]
                n159 = shared-variable "FOFB-Controller\\Actuation Network\\PS-RA01B\\User-Defined Variables\\ALV02A-Reading"(w251) -> ()  [unwired: 1 in, 1 out]
                n160 = shared-variable "FOFB-Controller\\Actuation Network\\PS-RA01B\\User-Defined Variables\\ALV02B-Reading"(w250) -> ()  [unwired: 1 in, 1 out]
                n161 = shared-variable "FOFB-Controller\\Actuation Network\\PS-RA01B\\User-Defined Variables\\ACH03A-Reading"(w249) -> ()  [unwired: 1 in, 1 out]
                n162 = shared-variable "FOFB-Controller\\Actuation Network\\PS-RA01B\\User-Defined Variables\\ACV03A-Reading"(w248) -> ()  [unwired: 1 in, 1 out]
                n163 = shared-variable "FOFB-Controller\\Actuation Network\\PS-RA01B\\User-Defined Variables\\ACH01B-Reading"(w247) -> ()  [unwired: 1 in, 1 out]
                n164 = shared-variable "FOFB-Controller\\Actuation Network\\PS-RA01B\\User-Defined Variables\\ACV01B-Reading"(w246) -> ()  [unwired: 1 in, 1 out]
                n165 = shared-variable "FOFB-Controller\\Actuation Network\\PS-RA01B\\User-Defined Variables\\PS-RA01B-Status"(w245) -> ()  [unwired: 1 in, 1 out]
              }
              frame condition #1 {
                n166 = shared-variable "FOFB-Controller\\Actuation Network\\PS-RA02B\\User-Defined Variables\\ACH04-Reading"(w261) -> ()  [unwired: 1 in, 1 out]
                n167 = shared-variable "FOFB-Controller\\Actuation Network\\PS-RA02B\\User-Defined Variables\\RRA02B-Reading"(w260) -> ()  [unwired: 1 in, 1 out]
                n168 = shared-variable "FOFB-Controller\\Actuation Network\\PS-RA02B\\User-Defined Variables\\ALV04A-Reading"(w259) -> ()  [unwired: 1 in, 1 out]
                n169 = shared-variable "FOFB-Controller\\Actuation Network\\PS-RA02B\\User-Defined Variables\\ALV04B-Reading"(w258) -> ()  [unwired: 1 in, 1 out]
                n170 = shared-variable "FOFB-Controller\\Actuation Network\\PS-RA02B\\User-Defined Variables\\ACH05A-Reading"(w257) -> ()  [unwired: 1 in, 1 out]
                n171 = shared-variable "FOFB-Controller\\Actuation Network\\PS-RA02B\\User-Defined Variables\\ACV05A-Reading"(w256) -> ()  [unwired: 1 in, 1 out]
                n172 = shared-variable "FOFB-Controller\\Actuation Network\\PS-RA02B\\User-Defined Variables\\ACH03B-Reading"(w255) -> ()  [unwired: 1 in, 1 out]
                n173 = shared-variable "FOFB-Controller\\Actuation Network\\PS-RA02B\\User-Defined Variables\\ACV03B-Reading"(w254) -> ()  [unwired: 1 in, 1 out]
                n174 = shared-variable "FOFB-Controller\\Actuation Network\\PS-RA02B\\User-Defined Variables\\PS-RA02B-Status"(w262) -> ()  [unwired: 1 in, 1 out]
              }
              frame condition #2 {
                n175 = shared-variable "FOFB-Controller\\Actuation Network\\PS-RA03B\\User-Defined Variables\\ACH06-Reading"(w270) -> ()  [unwired: 1 in, 1 out]
                n176 = shared-variable "FOFB-Controller\\Actuation Network\\PS-RA03B\\User-Defined Variables\\RRA03B-Reading"(w269) -> ()  [unwired: 1 in, 1 out]
                n177 = shared-variable "FOFB-Controller\\Actuation Network\\PS-RA03B\\User-Defined Variables\\ALV06A-Reading"(w268) -> ()  [unwired: 1 in, 1 out]
                n178 = shared-variable "FOFB-Controller\\Actuation Network\\PS-RA03B\\User-Defined Variables\\ALV06B-Reading"(w267) -> ()  [unwired: 1 in, 1 out]
                n179 = shared-variable "FOFB-Controller\\Actuation Network\\PS-RA03B\\User-Defined Variables\\ACH07A-Reading"(w266) -> ()  [unwired: 1 in, 1 out]
                n180 = shared-variable "FOFB-Controller\\Actuation Network\\PS-RA03B\\User-Defined Variables\\ACV07A-Reading"(w265) -> ()  [unwired: 1 in, 1 out]
                n181 = shared-variable "FOFB-Controller\\Actuation Network\\PS-RA03B\\User-Defined Variables\\ACH05B-Reading"(w264) -> ()  [unwired: 1 in, 1 out]
                n182 = shared-variable "FOFB-Controller\\Actuation Network\\PS-RA03B\\User-Defined Variables\\ACV05B-Reading"(w263) -> ()  [unwired: 1 in, 1 out]
                n183 = shared-variable "FOFB-Controller\\Actuation Network\\PS-RA03B\\User-Defined Variables\\PS-RA03B-Status"(w271) -> ()  [unwired: 1 in, 1 out]
              }
              frame condition #3 {
                n184 = shared-variable "FOFB-Controller\\Actuation Network\\PS-RA04B\\User-Defined Variables\\ACH08-Reading"(w279) -> ()  [unwired: 1 in, 1 out]
                n185 = shared-variable "FOFB-Controller\\Actuation Network\\PS-RA04B\\User-Defined Variables\\RRA04B-Reading"(w278) -> ()  [unwired: 1 in, 1 out]
                n186 = shared-variable "FOFB-Controller\\Actuation Network\\PS-RA04B\\User-Defined Variables\\ALV08A-Reading"(w277) -> ()  [unwired: 1 in, 1 out]
                n187 = shared-variable "FOFB-Controller\\Actuation Network\\PS-RA04B\\User-Defined Variables\\ALV08B-Reading"(w276) -> ()  [unwired: 1 in, 1 out]
                n188 = shared-variable "FOFB-Controller\\Actuation Network\\PS-RA04B\\User-Defined Variables\\ACH09A-Reading"(w275) -> ()  [unwired: 1 in, 1 out]
                n189 = shared-variable "FOFB-Controller\\Actuation Network\\PS-RA04B\\User-Defined Variables\\ACV09A-Reading"(w274) -> ()  [unwired: 1 in, 1 out]
                n190 = shared-variable "FOFB-Controller\\Actuation Network\\PS-RA04B\\User-Defined Variables\\ACH07B-Reading"(w273) -> ()  [unwired: 1 in, 1 out]
                n191 = shared-variable "FOFB-Controller\\Actuation Network\\PS-RA04B\\User-Defined Variables\\ACV07B-Reading"(w272) -> ()  [unwired: 1 in, 1 out]
                n192 = shared-variable "FOFB-Controller\\Actuation Network\\PS-RA04B\\User-Defined Variables\\PS-RA04B-Status"(w280) -> ()  [unwired: 1 in, 1 out]
              }
              frame condition #4 {
                n193 = shared-variable "FOFB-Controller\\Actuation Network\\PS-RA05B\\User-Defined Variables\\ACH10-Reading"(w288) -> ()  [unwired: 1 in, 1 out]
                n194 = shared-variable "FOFB-Controller\\Actuation Network\\PS-RA05B\\User-Defined Variables\\RRA05B-Reading"(w287) -> ()  [unwired: 1 in, 1 out]
                n195 = shared-variable "FOFB-Controller\\Actuation Network\\PS-RA05B\\User-Defined Variables\\ALV10A-Reading"(w286) -> ()  [unwired: 1 in, 1 out]
                n196 = shared-variable "FOFB-Controller\\Actuation Network\\PS-RA05B\\User-Defined Variables\\ALV10B-Reading"(w285) -> ()  [unwired: 1 in, 1 out]
                n197 = shared-variable "FOFB-Controller\\Actuation Network\\PS-RA05B\\User-Defined Variables\\ACH11A-Reading"(w284) -> ()  [unwired: 1 in, 1 out]
                n198 = shared-variable "FOFB-Controller\\Actuation Network\\PS-RA05B\\User-Defined Variables\\ACV11A-Reading"(w283) -> ()  [unwired: 1 in, 1 out]
                n199 = shared-variable "FOFB-Controller\\Actuation Network\\PS-RA05B\\User-Defined Variables\\ACH09B-Reading"(w282) -> ()  [unwired: 1 in, 1 out]
                n200 = shared-variable "FOFB-Controller\\Actuation Network\\PS-RA05B\\User-Defined Variables\\ACV09B-Reading"(w281) -> ()  [unwired: 1 in, 1 out]
                n201 = shared-variable "FOFB-Controller\\Actuation Network\\PS-RA05B\\User-Defined Variables\\PS-RA05B-Status"(w289) -> ()  [unwired: 1 in, 1 out]
              }
              frame condition #5 {
                n202 = shared-variable "FOFB-Controller\\Actuation Network\\PS-RA06B\\User-Defined Variables\\ACH12-Reading"(w297) -> ()  [unwired: 1 in, 1 out]
                n203 = shared-variable "FOFB-Controller\\Actuation Network\\PS-RA06B\\User-Defined Variables\\RRA06B-Reading"(w296) -> ()  [unwired: 1 in, 1 out]
                n204 = shared-variable "FOFB-Controller\\Actuation Network\\PS-RA06B\\User-Defined Variables\\ALV12A-Reading"(w295) -> ()  [unwired: 1 in, 1 out]
                n205 = shared-variable "FOFB-Controller\\Actuation Network\\PS-RA06B\\User-Defined Variables\\ALV12B-Reading"(w294) -> ()  [unwired: 1 in, 1 out]
                n206 = shared-variable "FOFB-Controller\\Actuation Network\\PS-RA06B\\User-Defined Variables\\ACH01A-Reading"(w293) -> ()  [unwired: 1 in, 1 out]
                n207 = shared-variable "FOFB-Controller\\Actuation Network\\PS-RA06B\\User-Defined Variables\\ACV01A-Reading"(w292) -> ()  [unwired: 1 in, 1 out]
                n208 = shared-variable "FOFB-Controller\\Actuation Network\\PS-RA06B\\User-Defined Variables\\ACH11B-Reading"(w291) -> ()  [unwired: 1 in, 1 out]
                n209 = shared-variable "FOFB-Controller\\Actuation Network\\PS-RA06B\\User-Defined Variables\\ACV11B-Reading"(w290) -> ()  [unwired: 1 in, 1 out]
                n210 = shared-variable "FOFB-Controller\\Actuation Network\\PS-RA06B\\User-Defined Variables\\PS-RA06B-Status"(w298) -> ()  [unwired: 1 in, 1 out]
              }
            }
          }
        }
      }
    }
  }
